vi "rtin_ControlGPIOMode.vi"(7 "Set":bool, 8 "error in":errorcluster, 10 "GPIOMode":i32, 11 "connection ID":refnum<k5>) -> (0 "error out":errorcluster, 2 "GPIOMode out":i32, 3 "connection ID":refnum<k5>)   [LabVIEW 2016]
doc: "Retrieves the GPIO mode for MIC Mode feature"
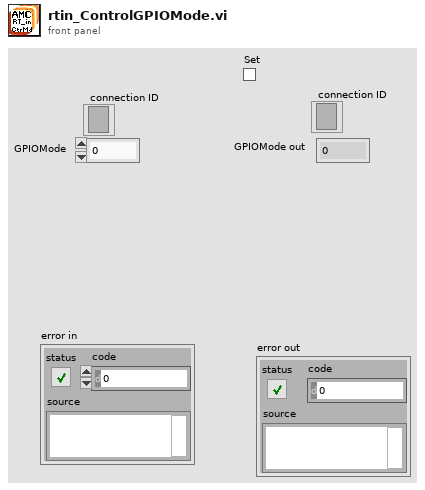
[diagram p1: front panel]
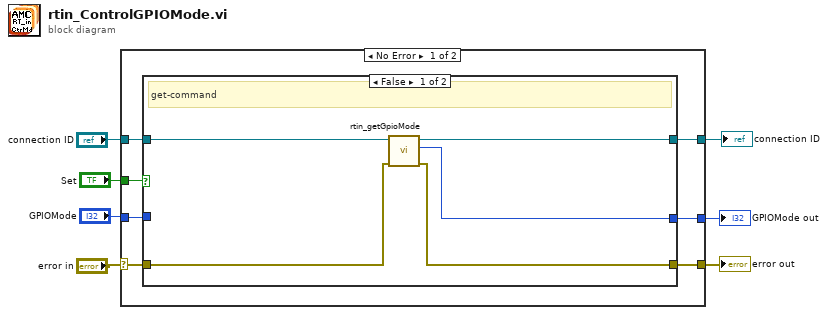
[diagram p0: block diagram]
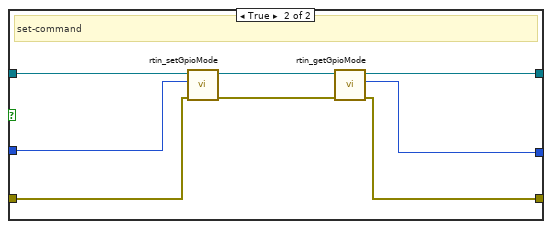
[diagram p2: hidden frame]
diagram:
  n1 = case shown="No Error" "error in" {
    selector: "error in" -> [w11 w30]
    tunnel: "GPIOMode" -> [w14 w28]
    tunnel: [w9 w30] -> w6
    tunnel: "Set" -> [w12 _]
    tunnel: [w10 w29] -> w4
    tunnel: "connection ID" -> [w13 w29]
    tunnel: [w8 w28] -> w1
    frame No Error {
      n2 = case shown="False" w12 {
        tunnel: w13 -> [w16 w26]
        tunnel: w14 -> [_ w21]
        tunnel: w11 -> [w19 w22]
        tunnel: [w17 w24] -> w10
        tunnel: [w18 w23] -> w9
        tunnel: [w15 w20] -> w8
        frame False {
          # "get-command"
          n3 = call "rtin_getGpioMode.vi"("error in"=w19, "connection ID"=w16) -> ("error out"=w18:errorcluster, "gpio_mode"=w15:i32, "connection ID"=w17:refnum<k5>)  [unwired: 7 in]
        }
        frame True {
          # "set-command"
          n4 = call "rtin_setGpioMode.vi"("error in"=w22, "gpio_mode"=w21, "connection ID"=w26) -> ("error out"=w27:errorcluster, "connection ID"=w25:refnum<k5>)  [unwired: 7 in]
          n5 = call "rtin_getGpioMode.vi"("error in"=w27, "connection ID"=w25) -> ("error out"=w23:errorcluster, "gpio_mode"=w20:i32, "connection ID"=w24:refnum<k5>)  [unwired: 7 in]
        }
      }
    }
    frame Error {
    }
  }
  "error out" <- w6
  "GPIOMode out" <- w1
  "connection ID" <- w4
